vi "GatedPulsesFid.vi"(1 "Gate":bool, 4 "Pulse bits":u64) -> ()   [LabVIEW 2019]
uses:
  <vilib>/rvi/eio/common/nirviEmuTemplateMethod_errors.vi
  <vilib>/eio/EIONode/EIONode.xnode
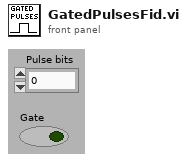
[diagram p1: front panel]
types:
  T1 = cluster{"Boolean array[0]":bool, "Boolean array[1]":bool, "Boolean array[2]":bool, "Boolean array[3]":bool, "Boolean array[4]":bool, "Boolean array[5]":bool, "Boolean array[6]":bool, "Boolean array[7]":bool, "Boolean array[8]":bool, "Boolean array[9]":bool, "Boolean array[10]":bool, "Boolean array[11]":bool, "Boolean array[12]":bool, "Boolean array[13]":bool, "Boolean array[14]":bool, "Boolean array[15]":bool, "Boolean array[16]":bool, "Boolean array[17]":bool, "Boolean array[18]":bool, "Boolean array[19]":bool, "Boolean array[20]":bool, "Boolean array[21]":bool, "Boolean array[22]":bool, "Boolean array[23]":bool, "Boolean array[24]":bool, "Boolean array[25]":bool, "Boolean array[26]":bool, "Boolean array[27]":bool, "Boolean array[28]":bool, "Boolean array[29]":bool, "Boolean array[30]":bool, "Boolean array[31]":bool, "Boolean array[32]":bool, "Boolean array[33]":bool, "Boolean array[34]":bool, "Boolean array[35]":bool, "Boolean array[36]":bool, "Boolean array[37]":bool, "Boolean array[38]":bool, "Boolean array[39]":bool}
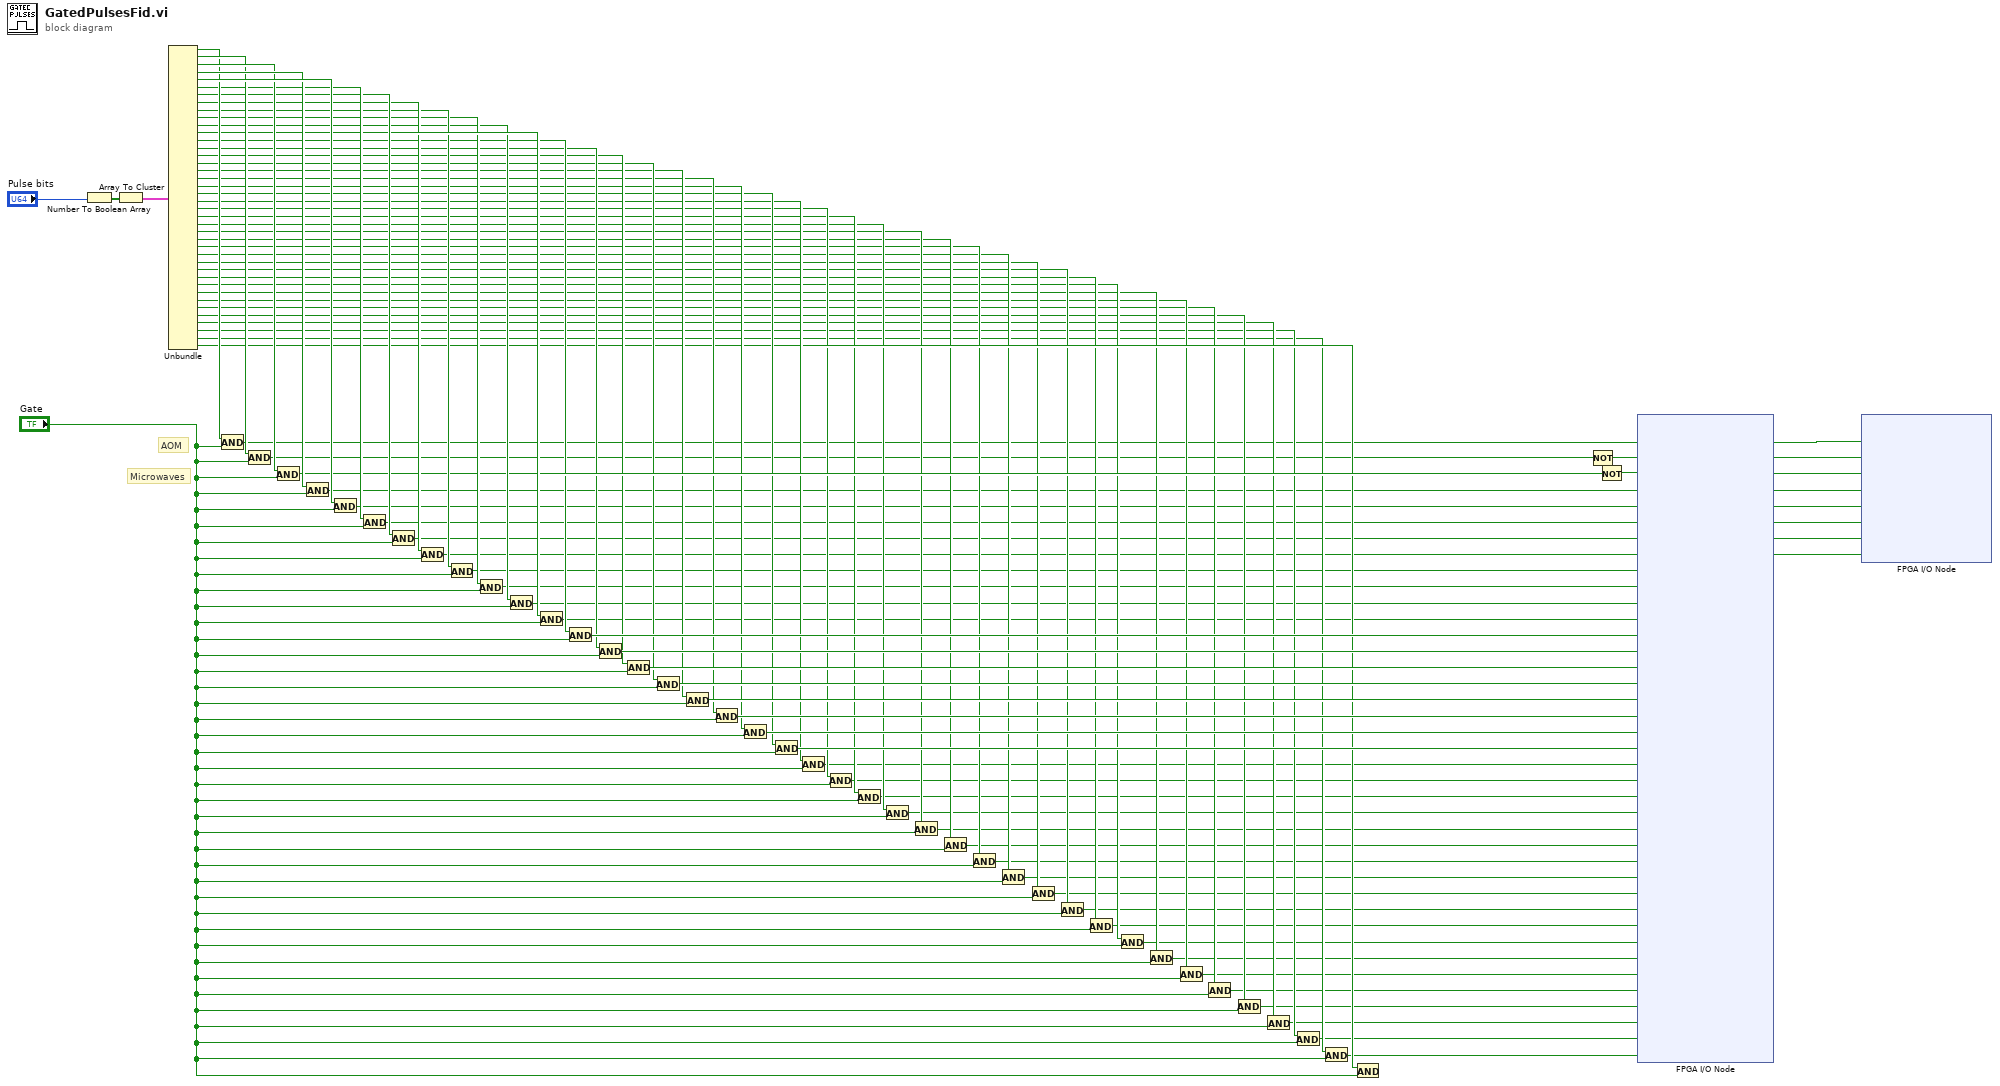
[diagram p0: block diagram]
diagram:
  # "Microwaves"
  # "AOM"
  n1 = Number To Boolean Array(number="Pulse bits") -> (Boolean array=w79:bool[])
  n2 = Array To Cluster(array=w79) -> (cluster=w80:T1)
  n3 = Unbundle(w80) -> ("Boolean array[0]"=w81:bool, "Boolean array[1]"=w82:bool, "Boolean array[2]"=w83:bool, "Boolean array[3]"=w84:bool, "Boolean array[4]"=w85:bool, "Boolean array[5]"=w77:bool, "Boolean array[6]"=w76:bool, "Boolean array[7]"=w74:bool, "Boolean array[8]"=w73:bool, "Boolean array[9]"=w72:bool, "Boolean array[10]"=w71:bool, "Boolean array[11]"=w75:bool, "Boolean array[12]"=w61:bool, "Boolean array[13]"=w60:bool, "Boolean array[14]"=w59:bool, "Boolean array[15]"=w58:bool, "Boolean array[16]"=w57:bool, "Boolean array[17]"=w56:bool, "Boolean array[18]"=w55:bool, "Boolean array[19]"=w54:bool, "Boolean array[20]"=w52:bool, "Boolean array[21]"=w50:bool, "Boolean array[22]"=w49:bool, "Boolean array[23]"=w48:bool, "Boolean array[24]"=w47:bool, "Boolean array[25]"=w46:bool, "Boolean array[26]"=w45:bool, "Boolean array[27]"=w44:bool, "Boolean array[28]"=w43:bool, "Boolean array[29]"=w42:bool, "Boolean array[30]"=w41:bool, "Boolean array[31]"=w40:bool, "Boolean array[32]"=w39:bool, "Boolean array[33]"=w38:bool, "Boolean array[34]"=w37:bool, "Boolean array[35]"=w36:bool, "Boolean array[36]"=w35:bool, "Boolean array[37]"=w34:bool, "Boolean array[38]"=w33:bool, "Boolean array[39]"=w51:bool)
  n4 = And(x=w81, y="Gate") -> (x .and. y?=w1:bool)
  n5 = And(x=w82, y="Gate") -> (x .and. y?=w13:bool)
  n6 = And(x=w83, y="Gate") -> (x .and. y?=w70:bool)
  n7 = And(x=w84, y="Gate") -> (x .and. y?=w11:bool)
  n8 = And(x=w85, y="Gate") -> (x .and. y?=w10:bool)
  n9 = And(x=w77, y="Gate") -> (x .and. y?=w9:bool)
  n10 = And(x=w76, y="Gate") -> (x .and. y?=w8:bool)
  n11 = And(x=w74, y="Gate") -> (x .and. y?=w7:bool)
  n12 = And(x=w73, y="Gate") -> (x .and. y?=w2:bool)
  n13 = And(x=w72, y="Gate") -> (x .and. y?=w6:bool)
  n14 = And(x=w71, y="Gate") -> (x .and. y?=w5:bool)
  n15 = And(x=w75, y="Gate") -> (x .and. y?=w4:bool)
  n16 = And(x=w61, y="Gate") -> (x .and. y?=w69:bool)
  n17 = And(x=w60, y="Gate") -> (x .and. y?=w68:bool)
  n18 = And(x=w59, y="Gate") -> (x .and. y?=w67:bool)
  n19 = And(x=w58, y="Gate") -> (x .and. y?=w66:bool)
  n20 = And(x=w57, y="Gate") -> (x .and. y?=w65:bool)
  n21 = And(x=w56, y="Gate") -> (x .and. y?=w64:bool)
  n22 = And(x=w55, y="Gate") -> (x .and. y?=w63:bool)
  n23 = And(x=w54, y="Gate") -> (x .and. y?=w62:bool)
  n24 = And(x=w52, y="Gate") -> (x .and. y?=w32:bool)
  n25 = And(x=w50, y="Gate") -> (x .and. y?=w31:bool)
  n26 = And(x=w49, y="Gate") -> (x .and. y?=w30:bool)
  n27 = And(x=w48, y="Gate") -> (x .and. y?=w29:bool)
  n28 = And(x=w47, y="Gate") -> (x .and. y?=w28:bool)
  n29 = And(x=w46, y="Gate") -> (x .and. y?=w27:bool)
  n30 = And(x=w45, y="Gate") -> (x .and. y?=w26:bool)
  n31 = And(x=w44, y="Gate") -> (x .and. y?=w25:bool)
  n32 = And(x=w43, y="Gate") -> (x .and. y?=w24:bool)
  n33 = And(x=w42, y="Gate") -> (x .and. y?=w23:bool)
  n34 = And(x=w41, y="Gate") -> (x .and. y?=w22:bool)
  n35 = And(x=w40, y="Gate") -> (x .and. y?=w21:bool)
  n36 = And(x=w39, y="Gate") -> (x .and. y?=w20:bool)
  n37 = And(x=w38, y="Gate") -> (x .and. y?=w19:bool)
  n38 = And(x=w37, y="Gate") -> (x .and. y?=w18:bool)
  n39 = And(x=w36, y="Gate") -> (x .and. y?=w17:bool)
  n40 = And(x=w35, y="Gate") -> (x .and. y?=w16:bool)
  n41 = And(x=w34, y="Gate") -> (x .and. y?=w15:bool)
  n42 = And(x=w33, y="Gate") -> (x .and. y?=w14:bool)
  n43 = And(x=w51, y="Gate") -> ()  [unwired: 1 out]
  n44 = Not(x=w13) -> (.not. x?=w3:bool)
  n45 = Not(x=w70) -> (.not. x?=w12:bool)
  n46 = xnode "FPGA I/O Node"("Connector1/DIO0"=w1, "Connector1/DIO1"=w3, "Connector1/DIO2"=w12, "Connector1/DIO3"=w11, "Connector1/DIO4"=w10, "Connector1/DIO5"=w9, "Connector1/DIO6"=w8, "Connector1/DIO7"=w7, "Connector1/DIO8"=w2, "Connector1/DIO9"=w6, "Connector1/DIO10"=w5, "Connector1/DIO11"=w4, "Connector1/DIO12"=w69, "Connector1/DIO13"=w68, "Connector1/DIO14"=w67, "Connector1/DIO15"=w66, "Connector1/DIO16"=w65, "Connector1/DIO17"=w64, "Connector1/DIO18"=w63, "Connector1/DIO19"=w62, "Connector1/DIO20"=w32, "Connector1/DIO21"=w31, "Connector1/DIO22"=w30, "Connector1/DIO23"=w29, "Connector1/DIO24"=w28, "Connector1/DIO25"=w27, "Connector1/DIO26"=w26, "Connector1/DIO27"=w25, "Connector1/DIO28"=w24, "Connector1/DIO29"=w23, "Connector1/DIO30"=w22, "Connector1/DIO31"=w21, "Connector1/DIO32"=w20, "Connector1/DIO33"=w19, "Connector1/DIO34"=w18, "Connector1/DIO35"=w17, "Connector1/DIO36"=w16, "Connector1/DIO37"=w15, "Connector1/DIO38"=w14) -> ()  [unwired: 39 in, 39 out]
  n47 = xnode "FPGA I/O Node"("Connector0/DIO0"=w1, "Connector0/DIO1"=w3, "Connector0/DIO2"=w12, "Connector0/DIO3"=w11, "Connector0/DIO4"=w10, "Connector0/DIO5"=w9, "Connector0/DIO6"=w8, "Connector0/DIO7"=w7) -> ()  [unwired: 8 in, 8 out]
